vi "To Camel Case (String)__ogtk.vi"(0 "string":string, 1 "no change if no spaces? (F=No)":bool) -> (2 "CamelCase string":string)   [LabVIEW 2014]
doc: "Converts alphabetic characters in string to \"camel\" case (i.e., first alphabetic character to uppercase, all others to lowercase for each \"word,\" removing spaces between words)."
uses:
  <userlib>/_OpenG.lib/string/string.llb/Trim Whitespace (String)__ogtk.vi
  <userlib>/_OpenG.lib/string/string.llb/To Proper Case (String Array)__ogtk.vi
panel:
  # "[OpenG VI Tags] ***Do Not Remove***"
  # "To Camel Case.vi\n\nConverts alphabetic characters in string to \"camel\" case (i.e., first alphabetic character to uppercase, all others to\nlowercase for each \"word,\" removing spaces between words).\n\nPlease visit http://www.OpenG.org to learn about the\nOpen Source LabVIEW software movement.\n\nNOTICE -- YOU MUST LEAVE THIS NOTICE IN PLACE.  PER THE TERMS OF THE LICENSE BELOW, YOU MAY SUBLICENSE THIS SOFTWARE \nIN ANY WAY THAT DOES NOT CONFLICT WITH THIS LICENSE.\n\n### BSD License (http://www.opensource.org/licenses/bsd-license.php) Begin ###\n \nCopyright (c) 2005, MKS Instruments, Inc., author: Doug Femec<doug_femec@mksinst.com>, IM dafemec\n\nAll rights reserved.\n\nRedistribution and use in source and binary forms, with or without modification, are permitted provided that the following conditions are met:\n\n    * Redistributions of source code must retain the above copyright notice, this list of conditions and the following disclaimer.\n    * Redistributions in binary form must reproduce the above copyright notice, this list of conditions and the following disclaimer in the \n       documentation and/or other materials provided with the distribution.\n    * Neither the name of SciWare, James Kring, Inc., nor the names of its contributors may be used to endorse or promote products derived \n       from this software without specific prior written permission.\n\nTHIS SOFTWARE IS PROVIDED BY THE COPYRIGHT HOLDERS AND CONTRIBUTORS \"AS IS\" AND ANY EXPRESS OR IMPLIED WARRANTIES, \nINCLUDING, BUT NOT LIMITED TO, THE IMPLIED WARRANTIES OF MERCHANTABILITY AND FITNESS FOR A PARTICULAR PURPOSE ARE \nDISCLAIMED. IN NO EVENT SHALL THE COPYRIGHT OWNER OR CONTRIBUTORS BE LIABLE FOR ANY DIRECT, INDIRECT, INCIDENTAL,\n SPECIAL, EXEMPLARY, OR CONSEQUENTIAL DAMAGES (INCLUDING, BUT NOT LIMITED TO, PROCUREMENT OF SUBSTITUTE GOODS OR \nSERVICES; LOSS OF USE, DATA, OR PROFITS; OR BUSINESS INTERRUPTION) HOWEVER CAUSED AND ON ANY THEORY OF LIABILITY, \nWHETHER IN CONTRACT, STRICT LIABILITY, OR TORT (INCLUDING NEGLIGENCE OR OTHERWISE) ARISING IN ANY WAY OUT OF THE USE \nOF THIS SOFTWARE, EVEN IF ADVISED OF THE POSSIBILITY OF SUCH DAMAGE.\n\n### BSD License End ###"
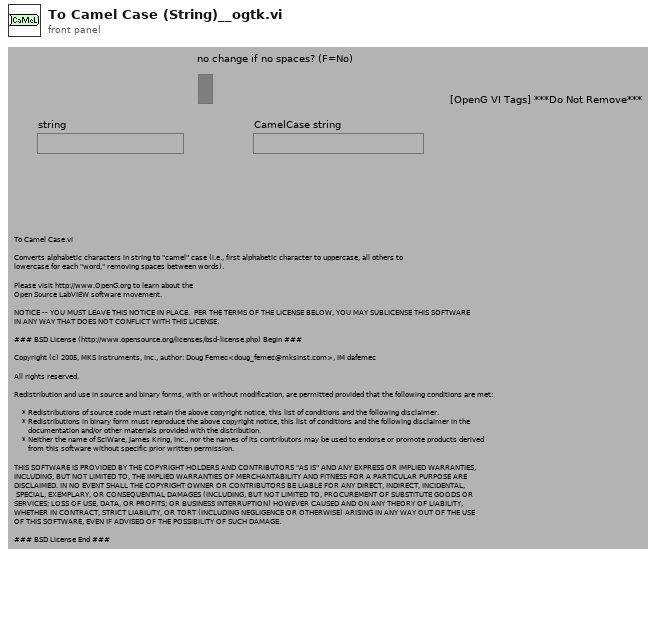
[diagram p1: front panel]
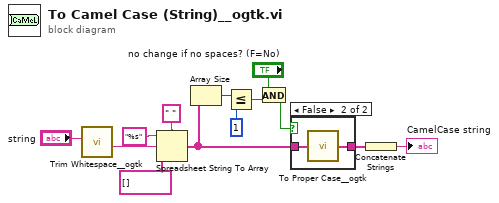
[diagram p0: block diagram]
diagram:
  n1 = call-poly <userlib>:"Trim Whitespace__ogtk.vi"("String in"="string") -> ("String out"=w12:string)  [unwired: 6 in]
  n2 = Spreadsheet String To Array(delimiter (Tab)=" ", format string="%s", spreadsheet string=w12, array type (2D Dbl)=string[] []) -> (array=w6:string[])
  n3 = Array Size(array=w6) -> (size(s)=w5:i32)
  n4 = Less Or Equal?(x=w5, y=1) -> (x <= y?=w3:bool)
  n5 = And(x="no change if no spaces? (F=No)", y=w3) -> (x .and. y?=w2:bool)
  n6 = case shown="False" w2 {
    tunnel: w6 -> [w14 w16]
    tunnel: [w14 w15] -> w8
    frame True {
    }
    frame False {
      n7 = call-poly <userlib>:"To Proper Case__ogtk.vi"("strings"=w16) -> ("proper case strings"=w15:string[])  [unwired: 4 in]
    }
  }
  n8 = Concatenate Strings(w8) -> (→"CamelCase string":string)
